vi "Pre Launch Init.vi"(11 "GameLogic in":refnum<class "GameLogic.lvclass">) -> (0 "error out":errorcluster, 3 "GameLogic out":refnum<class "GameLogic.lvclass">)   [LabVIEW 2019, in "GameLogic.lvlib" / "GameLogic.lvclass"]
doc: "(<B>Filename</B>: Actor Framework.lvlib:Actor.lvclass:Pre Launch Init.vi)\n\nDefines behavior that occurs after the Launch Nested Actor method is invoked but before the actor's Actor Core method begins running.\n\nBy default, this method does nothing. A descendant class may override it to define behavior."
uses:
  GameLogic.lvclass
  GameLogic.lvclass/GameLogic.ctl
  <vilib>/ActorFramework/Actor/Actor.lvclass
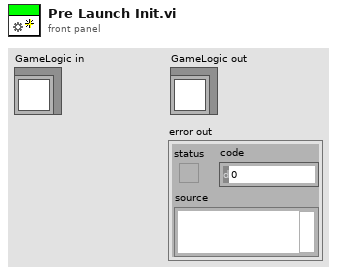
[diagram p1: front panel]
types:
  T1 = cluster{"Blue":bool, "Green":bool, "Red":bool, "Yellow":bool}
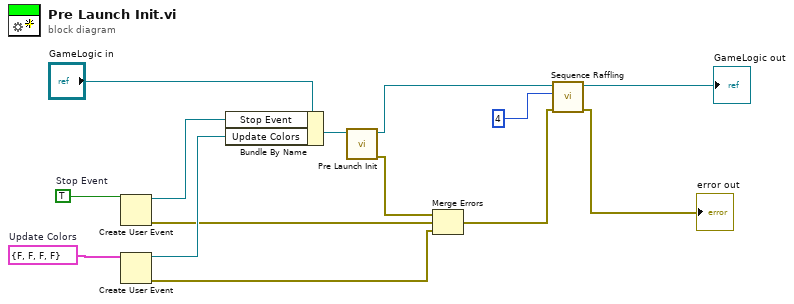
[diagram p0: block diagram]
diagram:
  w13 = T1 {"Blue"=FALSE, "Green"=FALSE, "Red"=FALSE, "Yellow"=FALSE}  # Update Colors
  w14 = TRUE  # Stop Event
  n1 = Create User Event(user event datatype=w14) -> (user event=w11:refnum<user-event>, error out=w8:errorcluster)  [unwired: 1 in]
  n2 = Create User Event(user event datatype=w13) -> (user event=w10:refnum<user-event>, error out=w6:errorcluster)  [unwired: 1 in]
  n3 = Bundle By Name(cluster="GameLogic in", "Stop Event"=w11, "Update Colors"=w10) -> (w9:refnum<class "GameLogic.lvclass">)
  n4 = call-parent "Pre Launch Init.vi"("Actor in"=w9) -> ("error out"=w7:errorcluster, "Actor out"=w4:refnum<class "GameLogic.lvclass">)  [unwired: 9 in]
  n5 = Merge Errors(w7, w8, w6) -> (w3:errorcluster)
  n6 = call "Sequence Raffling.vi"("error in (no error)"=w3, "Number of Raffles"=4, "GameLogic in"=w4) -> ("error out"=→"error out":errorcluster, "GameLogic out"=→"GameLogic out":refnum<class "GameLogic.lvclass">)  [unwired: 7 in]
